vi "GetAcqSeqGage.vi"(0 "Digitizer Settings":T5={"Digitizer delay (us) "=0.0, "rf points per line"=2048, "lines per plane"=128, "Samp Rate (Hz)"=100000000.0, "Additional dig delay (us)"=0.0, "Voltage Scale"=0.4, "Pre-Looks"=0, "Offset delay (us)"=0.0, "bits A/D"=8, "Avg Num"=1, "DigTimeOut"=5.0, "Rel Dig Delay"=0.0, "Dig Ch"=0, "LeCroyCluster"={"LeCroy Channels"=[TRUE, FALSE, FALSE, FALSE], "LC read pt offset"=0.0, "Sweep Avg"=FALSE}, "Main Digitizer"=enum."NI Digitizer", "Dig Config"=enum."Single channel", "Digitizer ID Cluster"={"Acqiris/Alazar/SP ID"=[], "NI Instr Handles"=[], "LeCroy VISA"="", "GaGe Handle"={"Handle"=0, "Sample size"=0, "Resolution"=0, "Offset"=0, "Channels"=0, "Boards"=0}, "ATS Ref"="ATS9350", "Acqiris Address"=["PCI::INSTR0"], "ADQRef"=refnum, "adq_cu_ptr"=refnum}, "Trigger Settings"={"Trig Source"=1, "Trig Coupling"=0, "Trig Slope"=0, "Level (mV)"=1500.0}, "Bulk Acq"=FALSE, "Bulk Start Indexes"=[], "Data Ref RF"=refnum, "NI ID/Channel"=[], "Total Dig CH"=1, "Xtra Ann Trig delay (us)"=10.0, "Fix Z Delay?"=FALSE, "One Way Transmission?"=FALSE, "Data Ref Log"=refnum} {"Trigger Settings"."Trig Slope" items=["Positive", "Negative"]; "Trigger Settings"."Level (mV)" format="%.2f"; "Trigger Settings"."Trig Coupling" items=["DC 1 MOhm", "AC 1 MOhm", "DC 50 Ohm", "AC 50 Ohm"]; "Trigger Settings"."Trig Source" items=["Chan 1", "External"]; "Rel Dig Delay" format="%.2f"; "DigTimeOut" format="%.2f"; "Avg Num" min=1; "Offset delay (us)" format="%.2f"; "Additional dig delay (us)" format="%.2f"; "Digitizer delay (us)" format="%.2f"}, 6 "Motion Settings":T1={"No Motion?"=FALSE, "Motion System"=enum."NI 735x", "Motion Bd ID"=1, "Motion Profile"="SMAC1", "# Axis"=1, "Reverse Z axis?"=TRUE, "SMAC Axis"=0, "scan pair"=enum."y-(x) scan", "RT fps"=6.0, "Steps per mm"=[1000, 1000, 1000, 1000], "Motor Parameters"={"velocity ct/s"=[10000.0, 10000.0, 10000.0, 50000.0], "accel ct/s^2"=[50000.0, 50000.0, 50000.0, 200000.0]}, "One Way Scan"=FALSE, "Reverse One Way Scan"=FALSE, "Global Position (mm)"=[], "Plane"=0, "Distance between\nscan lines (um)"=0.0, "Distance between\nscan planes (um)"=0.0, "number of scan planes"=1, "Total steps in line"=0, "Xtra plane\ndistance  (um)"=100, "Xtra planes "=1, "Add Axis"=FALSE, "overshoot cts"=200, "BKPT Shift"=0, "Scan Start Time (ms)"=0, "ESP VISA"="GPIB::1::INSTR", "3rd Axis"=1, "GL Ref Out"=refnum, "Galil Address"=""} {"3rd Axis" items=["x", "y", "z", "w"]; "Xtra planes" min=1; "Xtra plane\ndistance  (um)" min=0; "Distance between\nscan planes (um)" format="%.2f"; "Distance between\nscan lines (um)" format="%.2f"; "SMAC Axis" items=["None"=0, "Axis 1"=1, "Axis 2"=2, "Axis 3"=3, "Axis 4"=4, "Axis 5"=5, "Axis 6"=6, "Axis 7"=7, "Axis 8"=8, "Vector Space 1"=17, "Vector Space 2"=18, "Vector Space 3"=19, "Vector Space 4"=20]; "Motion Bd ID" min=1 max=32 step=1}, 8 "Numbered File":string, 10 "lines per plane":i32, 11 "Channel":u16(ring) items=["Channel 1", "Channel 2", "Channel 3", "Channel 4", "Memory 1", "Memory 2", "Memory 3", "Memory 4", "Function 1", "Function 2", "Function 3", "Function 4", "Function 5", "Function 6", "Function 7", "Function 8", "Other"], 14 "save?":bool=TRUE, 15 "Reverse?":bool) -> (17 "Raw VGain (scale)":dbl, 18 "Voltage Scale":T10, 20 "Array":i16[][](array[numeric]), 21 "VGain (dB)":dbl)   [LabVIEW 2022 SP3]
uses:
  -DigitizerRoutines/DigitizerSettings.ctl
  -DigitizerRoutines/DigitizerID.ctl
  -DigitizerRoutines/Digitizer.ctl
  Motion Controllers/NI_controller/-NI_MotionRoutines/MotionSys.ctl
  Motion Controllers/-MotionRoutines/ScanAxis.ctl
  Motion Controllers/NI_controller/-NI_MotionRoutines/MotionParameters.ctl
  -DigitizerRoutines/DigConfig.ctl
  Motion Controllers/-MotionRoutines/3rdAxis.ctl
  C:/Windows/System32/ADQAPI_dotNet_helper.dll
panel:
  out "Handle ClusterOut":T9
  in  "Timeout (10000 ms)":u32=10000
  # "1-D and 2-D B scan settings"
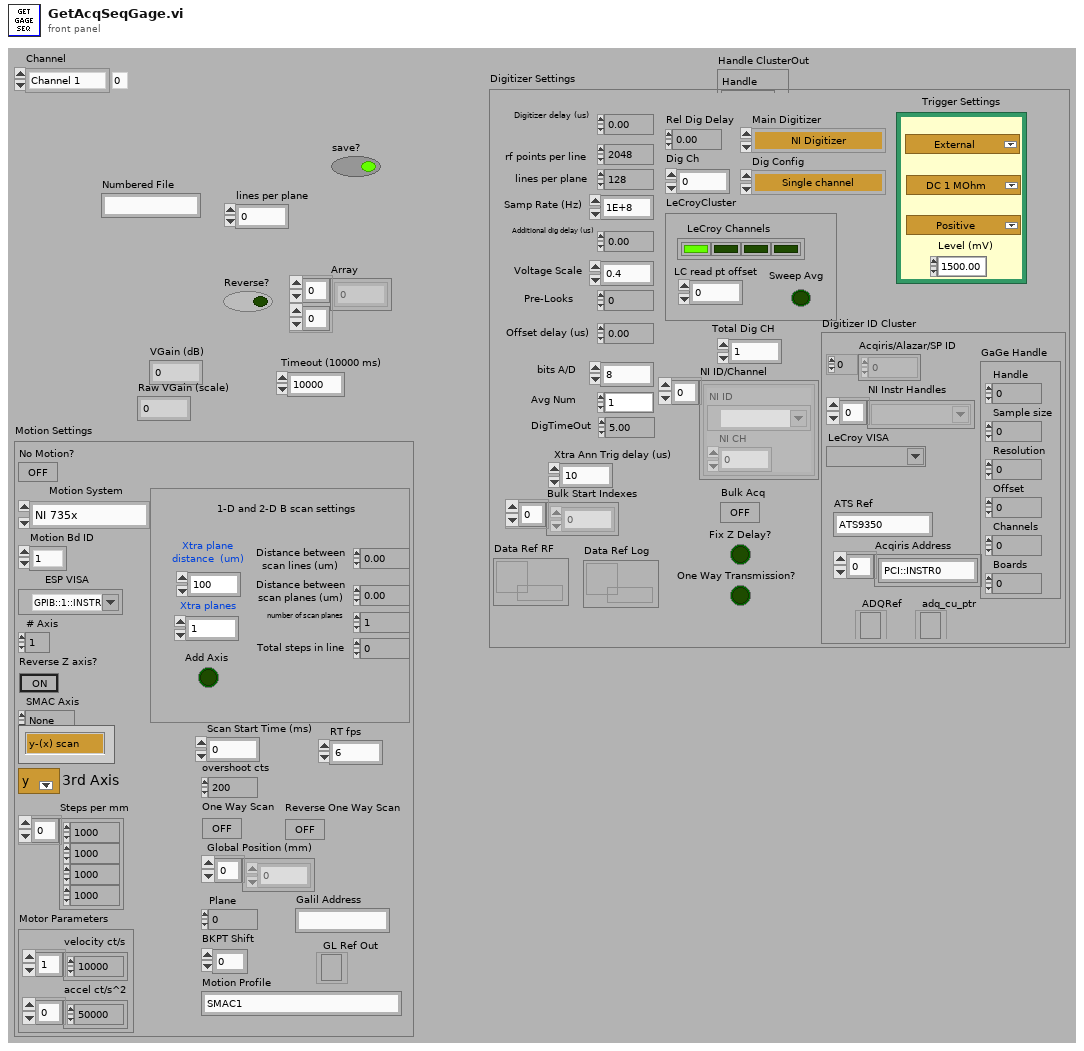
[diagram p1: front panel]
types:
  T1 = typedef "MotionParameters.ctl" = cluster{"No Motion?":bool, "Motion System":T2, "Motion Bd ID":u8, "Motion Profile":string, "# Axis":i8, "Reverse Z axis?":bool, "SMAC Axis":u16, "scan pair":T3, "RT fps":sgl, "Steps per mm":i32[], "Motor Parameters":cluster{"velocity ct/s":dbl[], "accel ct/s^2":dbl[]}, "One Way Scan":bool, "Reverse One Way Scan":bool, "Global Position (mm)":dbl[], "Plane":i32, "Distance between\nscan lines (um)":sgl, "Distance between\nscan planes (um)":sgl, "number of scan planes":i32, "Total steps in line":i32, "Xtra plane\ndistance  (um)":i32, "Xtra planes ":i32, "Add Axis":bool, "overshoot cts":i32, "BKPT Shift":i32, "Scan Start Time (ms)":u32, "ESP VISA":refnum<visa-resource-name>, "3rd Axis":T4, "GL Ref Out":refnum<k7>, "Galil Address":string}
  T2 = typedef "MotionSys.ctl" = enum16{"MM3000", "NI 735x", "Newport ESP", "No Motion Card", "Galil"}
  T3 = typedef "ScanAxis.ctl" = enum16{"y-(x) scan", "x-(y) scan", "z-(x) scan", "z-(y) scan", "y-(z) scan", "x-(z) scan", "w-(x) scan", "w-(y) scan", "w-(z) scan", "x-(w) scan", "y-(w) scan", "z-(w) scan"}
  T4 = typedef "3rdAxis.ctl" = u16
  T5 = typedef "DigitizerSettings.ctl" = cluster{"Digitizer delay (us) ":dbl, "rf points per line":i32, "lines per plane":i32, "Samp Rate (Hz)":dbl, "Additional dig delay (us)":dbl, "Voltage Scale":dbl, "Pre-Looks":i32, "Offset delay (us)":dbl, "bits A/D":i8, "Avg Num":i32, "DigTimeOut":sgl, "Rel Dig Delay":sgl, "Dig Ch":i32, "LeCroyCluster":cluster{"LeCroy Channels":bool[], "LC read pt offset":dbl, "Sweep Avg":bool}, "Main Digitizer":T6, "Dig Config":T7, "Digitizer ID Cluster":T8, "Trigger Settings":cluster{"Trig Source":u16, "Trig Coupling":u16, "Trig Slope":u16, "Level (mV)":dbl}, "Bulk Acq":bool, "Bulk Start Indexes":i32[], "Data Ref RF":refnum<data-value>, "NI ID/Channel":cluster{"NI ID":refnum<k15>, "NI CH":i32}[], "Total Dig CH":i32, "Xtra Ann Trig delay (us)":dbl, "Fix Z Delay?":bool, "One Way Transmission?":bool, "Data Ref Log":refnum<data-value>}
  T6 = typedef "Digitizer.ctl" = enum16{"Acqiris Digitizer", "NI Digitizer", "LeCroy", "GaGe", "AlazarTech", "No Digitizer", "Teledyne"}
  T7 = typedef "DigConfig.ctl" = enum16{"Single channel", "2 Chans w/ 2 Acqiris", "2 Chans w/ 1 Acqiris", "5-CH Pulser New", "5-CH pulser w/ ann array", "5-pass style ann array", "Empty"}
  T8 = typedef "DigitizerID.ctl" = cluster{"Acqiris/Alazar/SP ID":u32[], "NI Instr Handles":refnum<k15>[], "LeCroy VISA":refnum<visa-resource-name>, "GaGe Handle":cluster{"Handle":u32, "Sample size":u32, "Resolution":i32, "Offset":i32, "Channels":u32, "Boards":u32}, "ATS Ref":string, "Acqiris Address":string[], "ADQRef":refnum<k24>, "adq_cu_ptr":refnum<k24>}
  T9 = cluster{"Handle":u32, "Sample size":u32, "Resolution":i32, "Offset":i32, "Channels":u32, "Boards":u32}
  T10 = cluster{sgl, "Gain [dB]  ":sgl, "Atten (dB)":sgl}
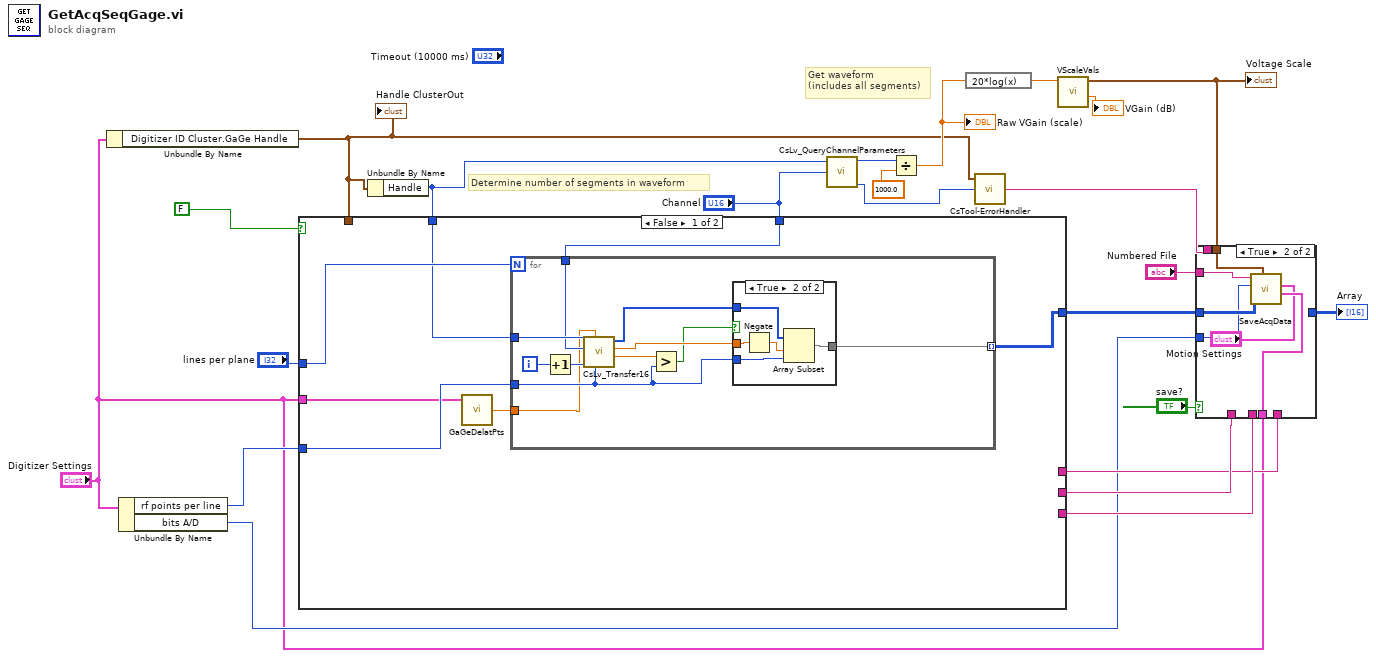
[diagram p0: block diagram]
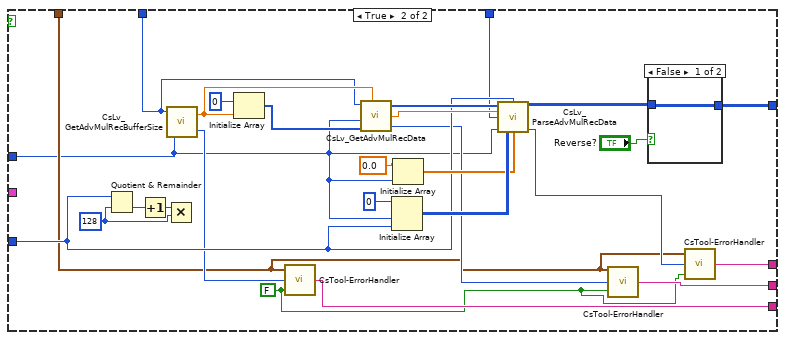
[diagram p3: hidden frame]
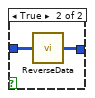
[diagram p4: hidden frame]
diagram:
  # "Determine number of segments in waveform"
  # "Get waveform\n(includes all segments)"
  n1 = Unbundle By Name("Digitizer Settings") -> ("Digitizer ID Cluster.GaGe Handle"=w4:T9)
  "Handle ClusterOut" <- w4
  n2 = Unbundle By Name("Digitizer Settings") -> ("rf points per line"=w3:i32, "bits A/D"=w2:i8)
  n3 = Unbundle By Name(w4) -> ("Handle"=w6:u32)
  n4 = case shown="False" FALSE {
    tunnel: [w27 w73] -> w21
    tunnel: w3 -> [w28 w59]
    tunnel: w4 -> [_ w55]
    tunnel: [_ w54] -> w16
    tunnel: [_ w53] -> w15
    tunnel: [_ w52] -> w14
    tunnel: "Channel" -> [w29 w50]
    tunnel: "lines per plane" -> [w30 w49]
    tunnel: w6 -> [w26 w48]
    tunnel: "Digitizer Settings" -> [w24 _]
    frame False {
      n5 = call "GaGeDelatPts.vi"("Digitizer Settings"=w24) -> ("Numeric"=w25:dbl)  [unwired: 4 in]
      n6 = for {
        N: w30 -> [_]
        tunnel: w29 -> [w38]
        tunnel: w28 -> [w40]
        tunnel: w26 -> [w41]
        tunnel: [w36] -> w27 mode=indexing
        tunnel: w25 -> [w34]
        i -> [w39]
        n7 = Increment(x=w39) -> (x+1=w35:i32)
        n8 = call <userlib>:"CsLv_Transfer16.vi"("Length (4096)"=w40, "Start (0)"=w34, "Segment (1)"=w35, "Channel (0)"=w38, "Handle"=w41) -> ("Actual Length"=w32:dbl, "Actual Start"=w33:dbl, "Buffer"=w37:i16[])  [unwired: 1 in, 1 out]
        n9 = Greater?(x=w32, y=w40) -> (0:w31:bool)
        n10 = case shown="True" w31 {
          tunnel: w37 -> [w42 w46]
          tunnel: [w42 w45] -> w36
          tunnel: w40 -> [_ w47]
          tunnel: w33 -> [_ w43]
          frame False {
          }
          frame True {
            n11 = Negate(x=w43) -> (-x=w44:dbl)
            n12 = Array Subset(array=w46, index=w44, length=w47) -> (w45:i16[])
          }
        }
      }
    }
    frame True {
      w51 = FALSE ("StopOnError (true)")
      w61 = 128
      n13 = Quotient & Remainder(x=w59, y=w61) -> (floor(x/y)=w60:i32)  [unwired: 1 out]
      n14 = Increment(x=w60) -> (x+1=w62:i32)
      n15 = Multiply(x=w62, y=w61) -> ()  [unwired: 1 out]
      n16 = call <userlib>:"CsLv_GetAdvMulRecBufferSize.vi"("Segment Count (1)"=w49, "Handle"=w48) -> ("Error Code"=w58:i32, "Size"=w68:dbl)  [unwired: 1 in]
      n17 = Initialize Array(i16 0, w68) -> (w70:i16[])
      n18 = call <userlib>:"CsTool-ErrorHandler.vi"("StopOnError (true)"=w51, "Error Code"=w58, "Handle Cluster"=w55) -> ("Error String"=w54:string)
      n19 = call <userlib>:"CsLv_GetAdvMulRecData.vi"("Handle"=w48, "Segment Count (1)"=w49, "Raw Buffer"=w70, "Size"=w68) -> ("Buffer"=w63:u8[], "Actual Size"=w67:dbl, "Error Code"=w57:i32)  [unwired: 1 in]
      n20 = Initialize Array(i16 0, w49, w59) -> (w66:i16[][])
      n21 = Initialize Array(0.0, w49) -> (w65:dbl[])
      n22 = call <userlib>:"CsLv_ParseAdvMulRecData.vi"("Raw Buffer"=w63, "Length"=w59, "Raw Buffer Size"=w67, "Channel (1)"=w50, "Segment Count"=w49, "Data Buffer"=w66, "Time Stamp Data"=w65) -> ("Data Buffer Out"=w64:i16[][], "Error Code"=w56:i32)  [unwired: 4 in, 3 out]
      n23 = call <userlib>:"CsTool-ErrorHandler.vi"("StopOnError (true)"=w51, "Error Code"=w57, "Handle Cluster"=w55) -> ("Error String"=w53:string)
      n24 = case shown="False" "Reverse?" {
        tunnel: w64 -> [w75 w77]
        tunnel: [w75 w76] -> w73
        frame False {
        }
        frame True {
          n25 = call "ReverseData.vi"("Array in"=w77) -> ("Array out"=w76:i16[][])
        }
      }
      n26 = call <userlib>:"CsTool-ErrorHandler.vi"("StopOnError (true)"=w51, "Error Code"=w56, "Handle Cluster"=w55) -> ("Error String"=w52:string)
    }
  }
  n27 = call <userlib>:"CsLv_QueryChannelParameters.vi"("Channel"="Channel", "Handle"=w6) -> ("Error Code"=w8:i32, "Input Range (mV)"=w12:u32)  [unwired: 5 out]
  n28 = Divide(x=w12, y=sgl 1000.0) -> (x/y=w10:sgl)
  "Raw VGain (scale)" <- w10
  n29 = expression code="20*log(x)"(w10) -> (w19:sgl)
  n30 = call <userlib>:"CsTool-ErrorHandler.vi"("Error Code"=w8, "Handle Cluster"=w4) -> ("Error String"=w7:string)  [unwired: 1 in]
  n31 = call "VScaleVals.vi"("Full Scale"=w19) -> ("vGain (dB)"=→"VGain (dB)":dbl, "Voltage Scale"=w18:T10)  [unwired: 8 in, 1 out]
  "Voltage Scale" <- w18
  n32 = case shown="True" "save?" {
    tunnel: w21 -> [w78 w84]
    tunnel: [w78 _] -> w20
    tunnel: "Numbered File" -> [_ w83]
    tunnel: w18 -> [_ w82]
    tunnel: w16 -> [_ _]
    tunnel: w15 -> [_ _]
    tunnel: w14 -> [_ _]
    tunnel: w7 -> [_ _]
    tunnel: w2 -> [_ w81]
    tunnel: "Digitizer Settings" -> [_ w80]
    frame False {
    }
    frame True {
      n33 = call "SaveAcqData.vi"("Digitizer Settings"=w80, "Motion Settings"="Motion Settings", "Votage scaling"=w82, "Array"=w84, "Dig Word Size"=w81, "File Name"=w83) -> ()  [unwired: 5 in]
    }
  }
  "Array" <- w20
